vi "bug C(T) exp start.vi"() -> ()   [LabVIEW 2019]
doc: "This is the Main VI for the bug C(T) experiment.\n\nIt allows the user to modify and verify the temperatures at which to measure the capacitance, the temperature control parameters and the waveform acquisition parameters at the beginning. It starts temperature control immediately upon being run.\n\nOnce in execution mode, it will attempt to measure the capacitance at each set point. When complete, it then allows the user to save the data to a file.\n\n It also allows the user to create a temperature log file that logs the temperature control details for each cycle during the experiment. This can be quite useful to analyze and refine the control parameters later on, or help understand why experiments might get off track in the middle of the night.\n\nPaul K Dixon\nP3600\nCSUSB Physics"
uses:
  components/typedefs/exp sequence.ctl
  components/typedefs/scale control.ctl
  components/typedefs/temp indicator.ctl
  components/typedefs/temp control status.ctl
  components/typedefs/PID control parameters.ctl
  components/typedefs/temp cont cluster.ctl
  components/typedefs/temp exec cluster.ctl
  components/typedefs/temp mode enum.ctl
  components/typedefs/temp cont utility.ctl
  components/typedefs/cap fit params.ctl
  components/typedefs/wvfm acq params.ctl
  components/typedefs/result.ctl
  components/typedefs/measurement.ctl
  components/globals/Bug globals.vi
panel:
  in  "wait (ms)":i32(slide)=200 scale=1.0..10000.0
  in  "update wait":bool
  in  "Monitor":T1(tab)=enum."System Status"
  in  "Scale Control":T2
  out "T cont status":T3={"Control status"=enum."In Settle Band", "Temp"=30.0, "Power"=0.0, "Time in settle band"=0.0, "Settled"=TRUE, "Low"=FALSE, "High"=FALSE, "Setpoint"=30.0, "Control"=TRUE, "In Settle Band"=TRUE} caption="Temperature Control Status" {"Setpoint" format="%_6g"; "Power" format="%_6g"; "Temp" format="%_6g"}
  out "Temperature Chart":T5(graph)={"temp out"=31.819617943507183, 30.0, 32.0, 28.0, 30.5, 29.5, 7.465816318676388}
  out "Manual Temp control":bool
  out "Setpoint (C)":dbl=30.0
  out "meas index":i32
  in  "clear chart":bool
  in  "dyn color":bool caption="dynamic background color"
  in  "Mod T cont":bool
  in  "mode":T6(tab)=enum."Capacitance vs Temp"
  out "temp path":path caption="temp log file path"
  out "logging temp":bool
  out "Temperature Graph":cluster{"t hist":dbl[], "T hist":dbl[]}[](graph)=[{"t hist"=[0.681, 1.01, 1.338, 1.667, 1.996, 2.323, 2.651, 2.979, 3.308, 3.636, 3.966, 4.294, 4.622, 4.95, 5.282, 5.614, 5.949, 6.292, 6.624, 6.956, 7.29, 7.629, 7.962, 8.298, 8.632, 8.961, 9.305, 9.649, 9.982, 10.321], "T hist"=[28.221637848568264, 28.335463471473247, 28.45177291236797, 28.578054212374127, 28.712611988419383, 28.84616557500516, 28.98818760788282, 29.12927903863408, 29.273265947327218, 29.420201611602806, 29.566232905582694, 29.70936480151545, 29.857453821818012, 29.996629768200933, 30.14076143529155, 30.28185384495856, 30.41983725429435, 30.556691662116748, 30.68413877422978, 30.810295121327613, 30.930958632049965, 31.052323535552546, 31.161736118199713, 31.269603761681765, 31.37376795546072, 31.474170088455764, 31.568601926879808, 31.65482002616045, 31.741394285589706, 31.819617943507183]}, {"t hist"=[0.681, 1.01, 1.338, 1.667, 1.996, 2.323, 2.651, 2.979, 3.308, 3.636, 3.966, 4.294, 4.622, 4.95, 5.282, 5.614, 5.949, 6.292, 6.624, 6.956, 7.29, 7.629, 7.962, 8.298, 8.632, 8.961, 9.305, 9.649, 9.982, 10.321], "T hist"=[61.64927318018057, 60.87935633362467, 59.91081367089514, 59.07163506893572, 58.05431280608125, 56.97210065484677, 55.985935993807566, 54.81990049342825, 53.76683173570311, 52.62763554543207, 51.438400944419776, 50.316274027152325, 49.20160602426924, 47.947916986672055, 46.929584951781365, 45.70234026722682, 44.56571400351665, 43.46069894631547, 42.34612964276051, 41.30873367322221, 40.22693480489379, 39.23489588337625, 38.167150974118684, 37.28797871837572, 36.32680632996466, 35.39340435832317, 34.47125846281813, 33.68091084957889, 32.922923294982894, 32.02199191964152]}]
  in  "show power":bool
  out "RC Graph":waveform(dbl)(graph) caption="RC Decay Graph"
  out "RC Fit":T7={"Resistance (Ohms)"=100000.0, "Est Time constant (s)"=0.0, "Est Capacitance (F)"=0.0} caption="RC Decay Fit"
  out "Temperature":dbl
  in  "index":u32 caption="Temp Index to View"
  out "N Meas":i32 caption="Number of Measurements"
  out "C vs T":cluster{dbl[], dbl[]}(graph) caption="Capacitance vs Temperature"
  out "C vs t":cluster{dbl[], dbl[]}(graph) caption="Capacitance vs Time"
  in  "status":T8(tab)
  out "Temp":T9={"T exec"={"T mode"=enum."Exit", "exec setpoint"=30.0, "reset"=FALSE, "man power"=0.5, "man"=FALSE, "log"=FALSE, "clear"=FALSE}, "T status"={"Control status"=enum."Below Control Band", "Temp"=30.0, "Power"=0.0, "Time in settle band"=0.0, "Settled"=FALSE, "Low"=FALSE, "High"=FALSE, "Setpoint"=30.0, "Control"=FALSE, "In Settle Band"=FALSE}, "T params"={"Setpoint"=30.0, "Control Bandwidth"=2.0, "Integral Time"=10.0, "Int\nON"=TRUE, "Derivative Tme"=0.2, "Der\nON"=TRUE, "Settle Bandwidth"=0.2, "Settle Time"=60.0}, "utility"={"meas index"=0, "wait (ms)"=300, "H Vmax"=8.5, "power out"=0.0, "heat volt out"=0.0, "heat volt in"=0.0, "therm volt"=0.0, "t T P hist"=[], "cont hist"=[]}} {"utility"."therm volt" format="%_6g"; "utility"."heat volt in" format="%_6g"; "utility"."heat volt out" format="%_6g"; "utility"."power out" format="%_6g"; "utility"."H Vmax" format="%_6g"; "T exec"."man power" format="%_6g"; "T exec"."exec setpoint" format="%_6g"; "T params"."Settle Time" step=1.0; "T params"."Settle Bandwidth" step=0.01; "T params"."Derivative Tme" step=0.01; "T params"."Integral Time" step=1.0; "T params"."Control Bandwidth" step=0.1; "T params"."Setpoint" step=0.1; "T status"."Setpoint" format="%_6g"; "T status"."Power" format="%_6g"; "T status"."Temp" format="%_6g"}
  out "meas":T14={"wvfm params"={"Num of avg"=100, "Num points"=1000, "Meas rate (Hz)"=100000.0}, "avg"={"t0"=timestamp(0 s since 1904-01-01), "dt"=1.0, "Y"=[]}, "raw wvfms"=[], "progress"={"avg done"=FALSE, "meas index"=0, "N waves"=100}, "t (s)"=0.0}
  out "results":T16[](array[typedef])
  out "x":bool caption="global exit"
  out "sec":bool caption="stop secondary loops"
  out "autosave":bool caption="autosave when complete"
  out "results SS":dbl[][](array[numeric]) caption="results spreadsheet" format="%#_3g"
  out "log temp":bool caption="logging temp"
  out "data file":path
  out "Exp Seq":T17 caption="Experimental Sequence"
  in  "setup":T18(tab)=enum."Experiment set up"
  out "T log file exists":bool
  out "T Cont Pars":T12={"Setpoint"=30.0, "Control Bandwidth"=2.0, "Integral Time"=10.0, "Int\nON"=TRUE, "Derivative Tme"=0.2, "Der\nON"=TRUE, "Settle Bandwidth"=0.2, "Settle Time"=60.0} caption="Temp Control Parameters" {"Settle Time" step=1.0; "Settle Bandwidth" step=0.01; "Derivative Tme" step=0.01; "Integral Time" step=1.0; "Control Bandwidth" step=0.1; "Setpoint" step=0.1}
  in  "set T params":bool
  in  "Default Set":dbl=30.0 caption="Default Setpoint (C)"
  out "temp log file path":path
  in  "create T log":bool
  in  "Header":string="This is a C(T) experiment being done in Physics 3600.\nIt records the decay response of an RC circuit where the capacitance is a strong function of temperature." caption="Header Comments"
  in  "create file":bool
  in  "wave params":T15={"Num of avg"=10, "Num points"=1000, "Meas rate (Hz)"=100000.0} caption="waveform parameters"
  out "Setpoints":dbl[](array[numeric])=[35.0, 40.0, 45.0] caption="Setpoint List"
  in  "mod set list":bool
  out "N Sets":i32=3 caption="Num of Setpoints"
  out "data file exists":bool
  out "data file":path
  in  "autosave":bool caption="autosave when complete"
  in  "min set t":dbl=20.0 caption="Min settle time (s)"
  out "init status":string caption="initialization status"
  in  "exit 2":bool
  in  "proceed":bool
  in  "imm meas":bool
  out "N Sets done":i32 caption="Setpoint Index"
  out "Curr Set":dbl=30.0 caption="Current Setpoint (C)"
  out "N Sets":i32 caption="Number of Setpoints"
  out "Set List":dbl[](array[numeric]) caption="Setpoint List"
  in  "early exit":bool
  out "N waves":i32 caption="Number of Waves"
  out "N done":i32 caption="Number Complete"
  out "Status":T19(ring) caption="Execution Status"
  out "Raw data":waveform(dbl)[](graph)
  out "total elapsed time (s)":i32
  out "Full Header":string caption="Header Comments in file"
  out "Data File":path
  in  "dont save":bool
  in  "save data":bool
  out "results":dbl[][](array[numeric]) format="%#_3g"
  in  "Hold Setpoint (C)":dbl=30.0
  out "total elapsed time (s)":i32
  in  "Manual Control":bool
  in  "Manual Power":dbl(slide) scale=0.0..1.0
  out "T data logging":bool caption="Temp data being logged"
  out "T Cont Params":T12={"Setpoint"=30.0, "Control Bandwidth"=2.0, "Integral Time"=10.0, "Int\nON"=TRUE, "Derivative Tme"=0.2, "Der\nON"=TRUE, "Settle Bandwidth"=0.2, "Settle Time"=60.0} caption="Temp Control Parameters" {"Settle Time" step=1.0; "Settle Bandwidth" step=0.01; "Derivative Tme" step=0.01; "Integral Time" step=1.0; "Control Bandwidth" step=0.1; "Setpoint" step=0.1}
  in  "exit":bool
  out "autosave 2":bool caption="Data Autosaved"
  # "Bug Experiment C(T) Measurement"
  # "Note that the primary Experimental Sequence TAB is \nunder system control, the others are under user control"
  # "Juan Gamez     \nP3600    \nCSUSB Physics"
  # "Temperature control starts\nimmediately upon start up\nat the default set point \nwith the default parameters"
  # "Experiment\nCompleted"
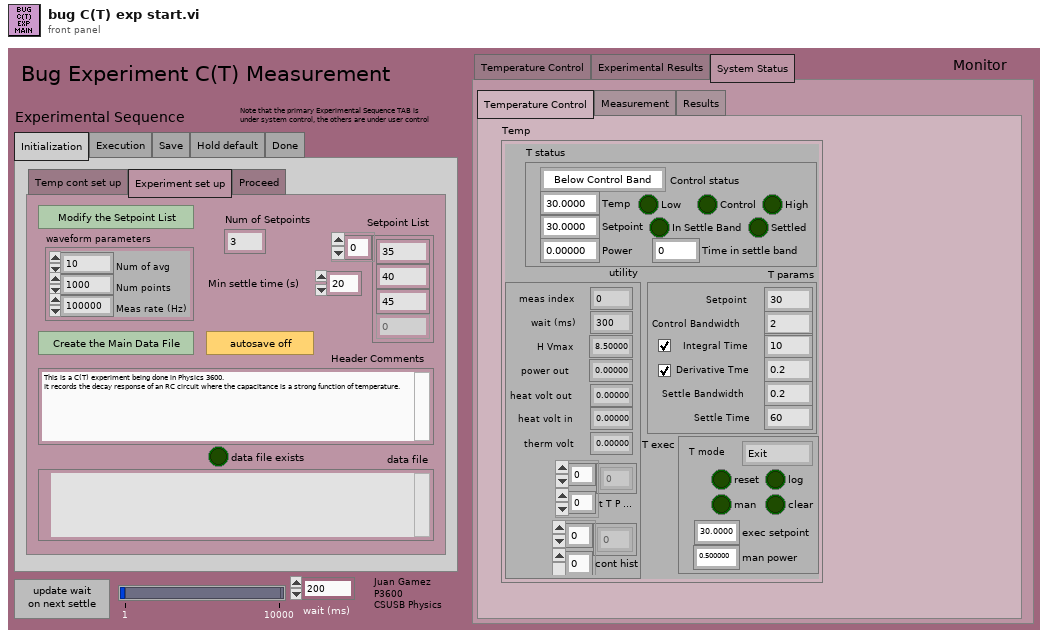
[diagram p1: front panel]
types:
  T1 = enum32{"Temperature Control", "Experimental Results", "System Status"}
  T2 = typedef "scale control.ctl" = cluster{"Full Scale":bool, "Control Scale":bool, "Settle Scale":bool, "Zoom Out X2":bool, "Zoom In X2":bool}
  T3 = typedef "temp indicator.ctl" = cluster{"Control status":T4, "Temp":dbl, "Power":dbl, "Time in settle band":dbl, "Settled":bool, "Low":bool, "High":bool, "Setpoint":dbl, "Control":bool, "In Settle Band":bool}
  T4 = typedef "temp control status.ctl" = enum16{"In Settle Band", "In Control Band", "Below Control Band", "Above Control Band"}
  T5 = cluster{"temp out":dbl, dbl, dbl, dbl, dbl, dbl, dbl}
  T6 = enum32{"Temperature overview", "RC decay graphs", "Capacitance vs Temp", "Capacitance vs Time"}
  T7 = typedef "cap fit params.ctl" = cluster{"Resistance (Ohms)":dbl, "Est Time constant (s)":dbl, "Est Capacitance (F)":dbl}
  T8 = enum32{"Temperature Control", "Measurement", "Results"}
  T9 = typedef "temp cont cluster.ctl" = cluster{"T exec":T10, "T status":T3, "T params":T12, "utility":T13}
  T10 = typedef "temp exec cluster.ctl" = cluster{"T mode":T11, "exec setpoint":dbl, "reset":bool, "man power":dbl, "man":bool, "log":bool, "clear":bool}
  T11 = typedef "temp mode enum.ctl" = enum16{"settling", "measuring", "holding", "Exit"}
  T12 = typedef "PID control parameters.ctl" = cluster{"Setpoint":dbl, "Control Bandwidth":dbl, "Integral Time":dbl, "Int\nON":bool, "Derivative Tme":dbl, "Der\nON":bool, "Settle Bandwidth":dbl, "Settle Time":dbl}
  T13 = typedef "temp cont utility.ctl" = cluster{"meas index":i32, "wait (ms)":i32, "H Vmax":dbl, "power out":dbl, "heat volt out":dbl, "heat volt in":dbl, "therm volt":dbl, "t T P hist":dbl[][], "cont hist":dbl[][]}
  T14 = typedef "measurement.ctl" = cluster{"wvfm params":T15, "avg":waveform(dbl), "raw wvfms":waveform(dbl)[], "progress":cluster{"avg done":bool, "meas index":i32, "N waves":i32}, "t (s)":dbl}
  T15 = typedef "wvfm acq params.ctl" = cluster{"Num of avg":i32, "Num points":i32, "Meas rate (Hz)":dbl}
  T16 = typedef "result.ctl" = cluster{"Temp (C)":dbl, "RC Fit":T7, "wave":waveform(dbl), "Time (s)":dbl}
  T17 = typedef "exp sequence.ctl" = enum32{"Initialization", "Execution", "Save", "Hold default", "Done"}
  T18 = enum32{"Temp cont set up", "Experiment set up", "Proceed"}
  T19 = enum16{"settling", "measuring", "holding", "Exit"}
  T20 = cluster{"temp out":dbl, dbl, dbl, dbl, dbl, dbl, dbl}[]
  T21 = typedef "DAQ state cluster.ctl" = cluster{"DAQ state":T22, "temp":T9, "meas":T14, "device":tag, "error":errorcluster, "start (ms)":i32}
  T22 = typedef "DAQ state enum.ctl" = enum16{"Global comm", "Meas T & P", "PID power calc", "Man Power set", "Output Power", "Wait", "Meas wvfm", "Avg wvfm", "Exit"}
  T23 = typedef "PID exec cluster.ctl" = cluster{"data file":T24, "T log file":T25, "exp seq":T26, "error":errorcluster}
  T24 = typedef "data file info.ctl" = cluster{"autosave":bool, "File refnum":refnum<file>, "data file path":path}
  T25 = typedef "bug temp file info.ctl" = cluster{"File refnum":refnum<file>, "T log file path":path, "exists":bool}
  T26 = typedef "exp seq cluster.ctl" = cluster{"wave params":T15, "Setpoints":dbl[], "#":i32, "index":i32, "elapsed time (s)":dbl, "set time (s)":dbl, "min settle (s)":dbl, " Exec Status":T27}
  T27 = typedef "bug meas status.ctl" = enum32{"Settling", "Measuring", "Holding", "Exit"}
  T28 = cluster{"Temp":dbl, "Setpoint":dbl, "THC":dbl, "TLC":dbl, "THS":dbl, "TLS":dbl, dbl}
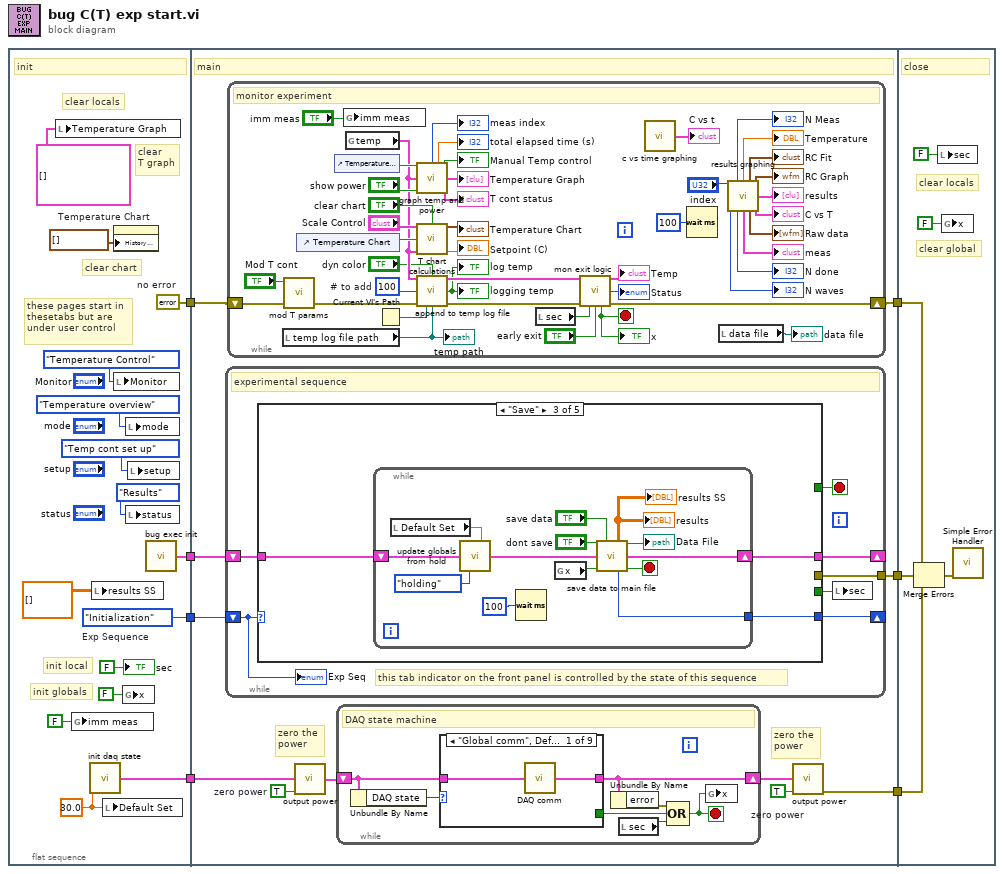
[diagram p0: block diagram]
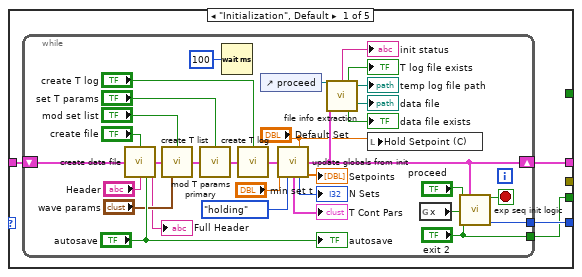
[diagram p2: hidden frame]
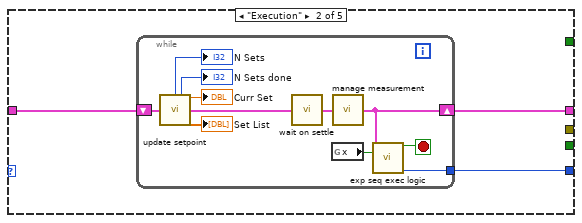
[diagram p3: hidden frame]
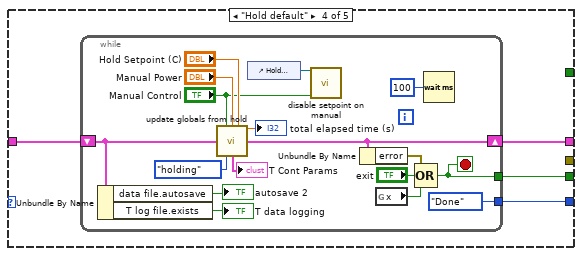
[diagram p4: hidden frame]
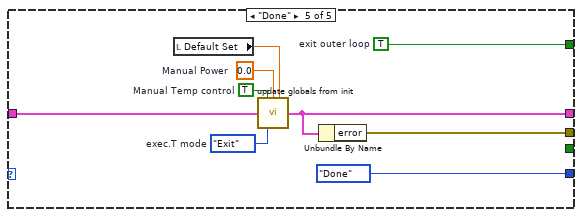
[diagram p5: hidden frame]
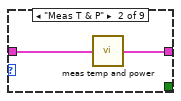
[diagram p6: hidden frame]
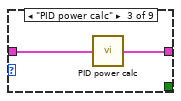
[diagram p7: hidden frame]
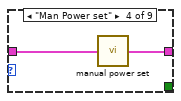
[diagram p8: hidden frame]
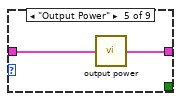
[diagram p9: hidden frame]
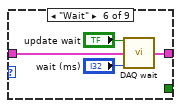
[diagram p10: hidden frame]
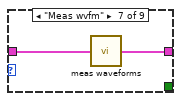
[diagram p11: hidden frame]
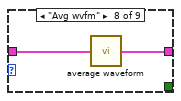
[diagram p12: hidden frame]
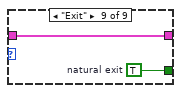
[diagram p13: hidden frame]
diagram:
  n1 = flat-sequence {
    tunnel: [w14] -> w6
    tunnel: [w20] -> w5
    tunnel: [w19] -> w2
    tunnel: [w18] -> w1
    tunnel: [w33] -> w7
    tunnel: w6 -> [w32]
    tunnel: w5 -> [w31]
    tunnel: [w28] -> w4
    tunnel: [w27] -> w3
    tunnel: w2 -> [w26]
    tunnel: w1 -> [w23]
    tunnel: w7 -> [w211]
    tunnel: w4 -> [w210]
    tunnel: w3 -> [w209]
    frame #0 {
      w18 = errorcluster {"status"=FALSE, "code"=0, "source"=""}  # no error
      w15 = 30.0 ("Default Set")
      w20 = exp_sequence."Initialization"  # Exp Sequence
      # "these pages start in \nthesetabs but are \nunder user control"
      # "init local"
      # "clear\nT graph"
      # "clear chart"
      # "clear locals"
      # "init globals"
      # "init"
      n2 = local write "Temperature Graph"(cluster{"t hist":dbl[], "T hist":dbl[]}[] [] ("Temperature Graph")) -> ()
      n3 = global write "Bug globals.vi" "imm meas"(FALSE ("imm meas")) -> ()
      n4 = call "init daq state.vi"("Default Setpoint (C)"=w15) -> ("DAQ clust out"=w19:T21)  [unwired: 14 in]
      n5 = local write "results SS"(dbl[][] [] ("saved results")) -> ()
      n6 = local write "Default Set"(w15) -> ()
      n7 = property on="Temperature Chart" class="WFChart (strict)"("History Data"=T20 []) -> ()  [unwired: 2 in, 2 out]
      n8 = local write "Monitor"(T1."Temperature Control" ("Monitor")) -> ()
      n9 = global write "Bug globals.vi" "x"(FALSE ("x")) -> ()
      n10 = local write "mode"(T6."Temperature overview" ("mode")) -> ()
      n11 = local write "status"(T8."Results" ("status")) -> ()
      n12 = local write "setup"(T18."Temp cont set up" ("setup")) -> ()
      n13 = call "bug exec init.vi"() -> ("exp exec"=w14:T23)  [unwired: 15 in]
      "sec" <- FALSE ("exit")
    }
    frame #1 {
      w25 = TRUE  # zero power
      w30 = TRUE  # zero power
      # "zero the \npower"
      # "zero the \npower"
      # "main"
      n14 = while {
        shift-right: [w81] -> _
        shift-left: w31 -> [w82]
        shift-right: [w83] -> _
        shift-left: w32 -> [w84]
        tunnel: [w79] -> w27
        stop <- w80 stop-if-true
        # "this tab indicator on the front panel is controlled by the state of this sequence"
        # "experimental sequence"
        n15 = case shown="\"Save\"" w82 {
          tunnel: w84 -> [w87 w122 w136 w153 w176]
          tunnel: [w88 w121 w135 w152 w175] -> w83
          tunnel: [w86 w123 w137 w151 exp_sequence."Done" ("Experimental Sequence")] -> w81
          tunnel: [_ _ _ _ w179] -> w80
          tunnel: [_ _ _ _ w177] -> w79
          tunnel: [w85 _ _ w150 _] -> w78
          frame "Initialization", Default {
            n16 = while {
              shift-right: [w98] -> w88
              shift-left: w87 -> [w111]
              tunnel: [w117] -> w86
              tunnel: ["exit 2"] -> w85
              stop <- w118 stop-if-true
              n17 = call "create data file.vi"("create file"="create file", "exp exec in"=w111, "Header"="Header", "autosave"="autosave") -> ("exp exec out"=w104:T23, "full \nheader"=→"Full Header":string)  [unwired: 10 in]
              n18 = call "create T list.vi"("mod set list"="mod set list", "exp exec in"=w104, "wave params"="wave params") -> ("exp exec out"=w103:T23)  [unwired: 10 in, 2 out]
              n19 = call "mod T params primary.vi"("Set T params"="set T params", "exp exec in"=w103) -> ("exp exec out"=w102:T23)  [unwired: 13 in]
              n20 = Wait (ms)(milliseconds to wait=u32 100) -> ()  [unwired: 1 out]
              n21 = call "create T log.vi"("create T log"="create T log", "exp exec in"=w102) -> ("exp exec out"=w110:T23)  [unwired: 12 in, 1 out]
              n22 = control-ref of="proceed"() -> (w94:refnum<vi>)
              n23 = call "update globals from init.vi"("Setpoint (C)"="Default Set", "exp exec in"=w110, "min set t"="min set t", "exec.T mode"=temp_mode_enum."holding") -> ("exp exec out"=w98:T23, "T params"=→"T Cont Pars":T12, "N Sets"=→"N Sets":i32, "Setpoints"=→"Setpoints":dbl[])  [unwired: 7 in, 1 out]
              n24 = call "file info extraction.vi"("proceed"=w94, "exp exec"=w98) -> ("message"=→"init status":string, "T log exists"=→"T log file exists":bool, "T log file"=→"temp log file path":path, "data file exists"=→"data file exists":bool, "data file"=→"data file":path)  [unwired: 9 in]
              n25 = local write "Hold Setpoint (C)"("Default Set") -> ()
              n26 = global read "Bug globals.vi" "x"() -> (w91:bool)
              n27 = call "exp seq init logic.vi"("proceed"="proceed", "exp exec in"=w98, "x"=w91, "exit"="exit 2") -> ("stop loop"=w118:bool, "Experimental Sequence"=w117:T17)  [unwired: 10 in]
              "autosave" <- "autosave"
            }
          }
          frame "Execution" {
            n28 = while {
              tunnel: [w134] -> w123
              shift-right: [w125] -> w121
              shift-left: w122 -> [w133]
              stop <- w124 stop-if-true
              n29 = call "update setpoint.vi"("exp exec in"=w133) -> ("Num set points"=→"N Sets":i32, "current setpoint index"=→"N Sets done":i32, "current set point"=→"Curr Set":dbl, "exp exec out"=w132:T23, "Setpoints"=→"Set List":dbl[])  [unwired: 10 in]
              n30 = call "wait on settle.vi"("exp exec in"=w132) -> ("exp exec out"=w131:T23)  [unwired: 14 in]
              n31 = global read "Bug globals.vi" "x"() -> (w126:bool)
              n32 = call "manage measurement.vi"("exp exec in"=w131) -> ("exp exec out"=w125:T23)  [unwired: 14 in]
              n33 = call "exp seq exec logic.vi"("exp exec"=w125, "x"=w126) -> ("exit"=w124:bool, "Experimental Sequence"=w134:T17)  [unwired: 12 in]
            }
          }
          frame "Save" {
            n34 = while {
              tunnel: [w149] -> w137
              shift-right: [w142] -> w135
              shift-left: w136 -> [w143]
              stop <- w144 stop-if-true
              n35 = local read "Default Set"() -> (w140:dbl)
              n36 = call "update globals from hold.vi"("Setpoint (C)"=w140, "exp exec in"=w143, "exec.T mode"=temp_mode_enum."holding") -> ("exp exec out"=w142:T23)  [unwired: 8 in, 4 out]
              n37 = Wait (ms)(milliseconds to wait=u32 100) -> ()  [unwired: 1 out]
              n38 = global read "Bug globals.vi" "x"() -> (w139:bool)
              n39 = call "save data to main file.vi"("dont save"="dont save", "save data"="save data", "exp exec in"=w142, "primary"=w139) -> ("results"=→"results" →"results SS":dbl[][], "data file path"=→"Data File":path, "Experimental Sequence"=w149:T17, "stop"=w144:bool)  [unwired: 7 in, 1 out]
            }
          }
          frame "Hold default" {
            n40 = while {
              shift-right: [w161] -> w152
              shift-left: w153 -> [w155]
              tunnel: [w163] -> w150
              tunnel: [exp_sequence."Done" ("Experimental Sequence")] -> w151
              stop <- w163 stop-if-true
              n41 = Unbundle By Name(w155) -> ("data file.autosave"=→"autosave 2":bool, "T log file.exists"=→"T data logging":bool)
              n42 = call "update globals from hold.vi"("Manual Temp control"="Manual Control", "Manual Power"="Manual Power", "Setpoint (C)"="Hold Setpoint (C)", "exp exec in"=w155, "exec.T mode"=temp_mode_enum."holding") -> ("Total elapsed time (s)"=→"total elapsed time (s)":dbl, "exp exec out"=w161:T23, "T params"=→"T Cont Params":T12)  [unwired: 6 in, 2 out]
              n43 = control-ref of="Hold Setpoint (C)"() -> (w166:refnum<vi>)
              n44 = call "disable setpoint on manual.vi"("Setpoint refnum"=w166, "Manual Control"="Manual Control") -> ()  [unwired: 14 in]
              n45 = Unbundle By Name(w161) -> ("error"=w162:errorcluster)
              n46 = global read "Bug globals.vi" "x"() -> (w154:bool)
              n47 = Compound Arithmetic op=OR(w162, "exit", w154) -> (w163:bool)
              n48 = Wait (ms)(milliseconds to wait=u32 100) -> ()  [unwired: 1 out]
            }
          }
          frame "Done" {
            w172 = TRUE  # Manual Temp control
            w173 = 0.0  # Manual Power
            w171 = temp_mode_enum."Exit"  # exec.T mode
            w179 = TRUE  # exit outer loop
            n49 = local read "Default Set"() -> (w174:dbl)
            n50 = call "update globals from init.vi"("Manual Temp control"=w172, "Manual Power"=w173, "Setpoint (C)"=w174, "exp exec in"=w176, "exec.T mode"=w171) -> ("exp exec out"=w175:T23)  [unwired: 6 in, 4 out]
            n51 = Unbundle By Name(w175) -> ("error"=w177:errorcluster)
          }
        }
        n52 = local write "sec"(w78) -> ()
        "Exp Seq" <- w82
      }
      n53 = while {
        shift-right: [w40] -> w33
        shift-left: w23 -> [w43]
        stop <- w48 stop-if-true
        w51 = 100  # # to add
        # "monitor experiment"
        n54 = local read "temp log file path"() -> (w75:path)
        "temp path" <- w75
        n55 = call "mod T params.vi"("Set T params"="Mod T cont", "error in (no error)"=w43) -> ("error out"=w42:errorcluster)  [unwired: 13 in]
        n56 = control-ref of="Temperature Chart"() -> (w67:refnum<vi>)
        n57 = control-ref of="Temperature Graph"() -> (w68:refnum<vi>)
        n58 = global write "Bug globals.vi" "imm meas"("imm meas") -> ()
        n59 = global read "Bug globals.vi" "temp"() -> (w54:T9)
        n60 = Current VI's Path() -> (path=w49:path)
        n61 = call "graph temp and power.vi"("Temperature Graph"=w68, "temp"=w54, "show power"="show power") -> ("meas index"=→"meas index":i32, "latest time (s)"=→"total elapsed time (s)":dbl, "man"=→"Manual Temp control":bool, "T and P graph"=→"Temperature Graph":cluster{"t hist":dbl[], "T hist":dbl[]}[], "T status"=→"T cont status":T3)  [unwired: 8 in]
        n62 = call "T chart calculations.vi"("Scale Control"="Scale Control", "clear chart"="clear chart", "WaveformChart in"=w67, "T cont"=w54) -> ("T chart cluster"=→"Temperature Chart":T28, "Setpoint"=→"Setpoint (C)":dbl)  [unwired: 10 in]
        n63 = call "append to temp log file.vi"("T cont"=w54, "dynamic color"="dyn color", "# to add"=w51, "error in (no error)"=w42, "main vi path"=w49, "temp log file path"=w75) -> ("T cont out"=w53:T9, "log exists"=→"logging temp" →"log temp":bool, "error out"=w55:errorcluster)  [unwired: 7 in]
        n64 = local read "sec"() -> (w38:bool)
        n65 = call "mon exit logic.vi"("temp"=w53, "error in (no error)"=w55, "sec"=w38, "early exit"="early exit") -> ("temp out"=→"Temp":T9, "T mode"=→"Status":T11, "exit loop"=w48:bool, "error out"=w40:errorcluster)  [unwired: 8 in]
        "x" <- w48
        n66 = call "c vs time graphing.vi"() -> ("C vs time graph"=→"C vs t":cluster{dbl[], dbl[]})  [unwired: 15 in]
        n67 = Wait (ms)(milliseconds to wait=u32 100) -> ()  [unwired: 1 out]
        n68 = local read "data file"() -> (→"data file":path)
        n69 = call "results graphing.vi"("set to view"="index") -> ("N Meas"=→"N Meas":i32, "Temperature"=→"Temperature":dbl, "RC Fit"=→"RC Fit":T7, "RC Graph"=→"RC Graph":waveform(dbl), "results out"=→"results":T16[], "N waves"=→"N waves":i32, "N done"=→"N done":i32, "meas"=→"meas":T14, "raw wvfms"=→"Raw data":waveform(dbl)[], "C vs T graph"=→"C vs T":cluster{dbl[], dbl[]})  [unwired: 5 in]
      }
      n70 = call "output power.vi"("DAQ cluster in"=w26, "zero power"=w25) -> ("DAQ cluster out"=w24:T21)  [unwired: 12 in, 1 out]
      n71 = while {
        shift-right: [w182] -> w29
        shift-left: w24 -> [w183]
        stop <- w180 stop-if-true
        # "DAQ state machine"
        n72 = Unbundle By Name(w183) -> ("DAQ state"=w184:T22)
        n73 = case shown="\"Global comm\", Default" w184 {
          tunnel: [_ _ _ _ _ _ _ _ w206] -> w185
          tunnel: w183 -> [w188 w190 w192 w194 w196 w200 w202 w204 w205]
          tunnel: [w187 w189 w191 w193 w195 w199 w201 w203 w205] -> w182
          frame "Global comm", Default {
            n74 = call "DAQ comm.vi"("DAQ cluster in"=w188) -> ("DAQ cluster out"=w187:T21)  [unwired: 14 in]
          }
          frame "Meas T & P" {
            n75 = call "meas temp and power.vi"("DAQ cluster in"=w190) -> ("DAQ cluster out"=w189:T21)  [unwired: 14 in]
          }
          frame "PID power calc" {
            n76 = call "PID power calc.vi"("DAQq cluster in"=w192) -> ("DAQ cluster out"=w191:T21)  [unwired: 14 in]
          }
          frame "Man Power set" {
            n77 = call "manual power set.vi"("DAQ cluster in"=w194) -> ("DAQ cluster out"=w193:T21)  [unwired: 14 in]
          }
          frame "Output Power" {
            n78 = call "output power.vi"("DAQ cluster in"=w196) -> ("DAQ cluster out"=w195:T21)  [unwired: 13 in, 1 out]
          }
          frame "Wait" {
            n79 = call "DAQ wait.vi"("update wait"="update wait", "DAQ cluster in"=w200, "wait (ms)"="wait (ms)") -> ("DAQ cluster out"=w199:T21)  [unwired: 12 in]
          }
          frame "Meas wvfm" {
            n80 = call "meas waveforms.vi"("DAQ cluster in"=w202) -> ("DAQ cluster out"=w201:T21)  [unwired: 14 in]
          }
          frame "Avg wvfm" {
            n81 = call "average waveform.vi"("DAQ cluster in"=w204) -> ("DAQ cluster out"=w203:T21)  [unwired: 14 in]
          }
          frame "Exit" {
            w206 = TRUE  # natural exit
          }
        }
        n82 = Unbundle By Name(w182) -> ("error"=w186:errorcluster)
        n83 = local read "sec"() -> (w181:bool)
        n84 = Compound Arithmetic op=OR(w186, w185, w181) -> (w180:bool)
        n85 = global write "Bug globals.vi" "x"(w180) -> ()
      }
      n86 = call "output power.vi"("DAQ cluster in"=w29, "zero power"=w30) -> ("error out"=w28:errorcluster)  [unwired: 12 in, 1 out]
    }
    frame #2 {
      # "clear global"
      # "clear locals"
      # "close"
      n87 = Merge Errors(w211, w209, w210) -> (w212:errorcluster)
      n88 = local write "sec"(FALSE ("exit")) -> ()
      n89 = global write "Bug globals.vi" "x"(FALSE ("x")) -> ()
      n90 = call <vilib>:"Simple Error Handler.vi"("error in (no error)"=w212) -> ()  [unwired: 4 in, 5 out]
    }
  }
